vi "Setup subWorker - subWorker 02.vi"(8 "error in":errorcluster, 11 "subWorker Level 1 in":refnum<class "subWorker Level 1.lvclass">) -> (0 "error out":errorcluster, 3 "subWorker Level 1 out":refnum<class "subWorker Level 1.lvclass">)   [LabVIEW 2017, in "subWorker Level 1.lvclass"]
doc: "This VI sets up the framework parameters of a statically-linked subWorker."
uses:
  subWorker Level 1.lvclass
  subWorker Level 1.lvclass/subWorker Level 1.ctl
  subWorker Level 2/subWorker Level 2.lvclass
  C:/Program Files (x86)/National Instruments/LabVIEW 2017/vi.lib/addons/_Workers/Library/Classes/Worker/Worker.lvclass
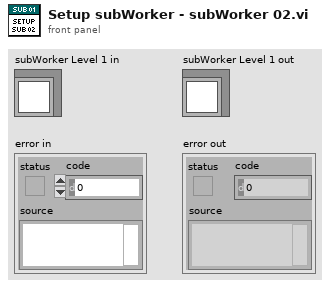
[diagram p1: front panel]
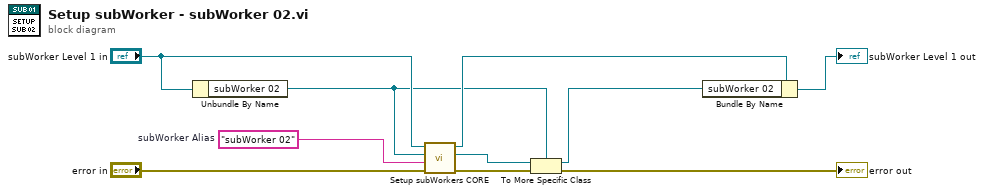
[diagram p0: block diagram]
diagram:
  w6 = "subWorker 02"  # subWorker Alias
  n1 = Unbundle By Name("subWorker Level 1 in") -> ("subWorker 02"=w3:refnum<class "subWorker Level 2.lvclass">)
  n2 = call-dynamic "Setup subWorkers CORE.vi"("error in"="error in", "subWorker Alias"=w6, "subWorker"=w3, "Worker"="subWorker Level 1 in") -> ("error out"=w5:errorcluster, "subWorker out"=w1:refnum<class "Worker.lvclass">, "Worker out"=w8:refnum<class "subWorker Level 1.lvclass">)  [unwired: 5 in]
  n3 = To More Specific Class(target class=w3, reference=w1, error in=w5) -> (specific class reference=w2:refnum<class "subWorker Level 2.lvclass">, error out=→"error out":errorcluster)
  n4 = Bundle By Name(cluster=w8, "subWorker 02"=w2) -> (→"subWorker Level 1 out":refnum<class "subWorker Level 1.lvclass">)
